vi "Destroy.vi"(0 "Dashboard Server in":refnum<class "Dashboard Server.lvclass">, 5 "error in (no error)":errorcluster) -> (14 "Dashboard Server out":refnum<class "Dashboard Server.lvclass">, 19 "error out":errorcluster)   [LabVIEW 2016, in "Dashboard Server.lvclass"]
uses:
  Dashboard Server.lvclass
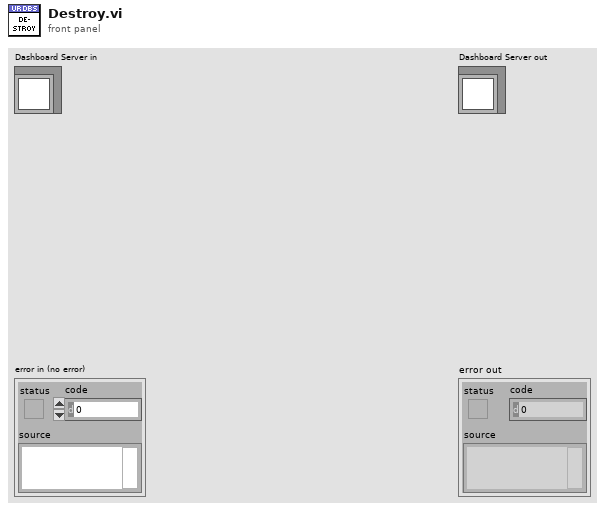
[diagram p1: front panel]
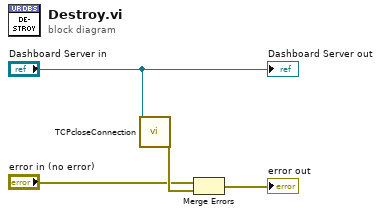
[diagram p0: block diagram]
diagram:
  n1 = call-dynamic "TCPcloseConnection.vi"("DashboardServer in"="Dashboard Server in") -> ("error out"=w3:errorcluster)  [unwired: 17 in, 1 out]
  n2 = Merge Errors("error in (no error)", w3) -> (→"error out":errorcluster)
  "Dashboard Server out" <- "Dashboard Server in"
